vi "Initialize.vi"(8 "error in (no error)":errorcluster, 11 "Socket in":refnum<class "Socket.lvclass">) -> (0 "error out":errorcluster, 3 "Socket out":refnum<class "Socket.lvclass">)   [LabVIEW 2018, in "Socket.lvclass"]
uses:
  Socket.lvclass
  Socket.lvclass/Socket.ctl
  State Machine/State Machine.lvclass
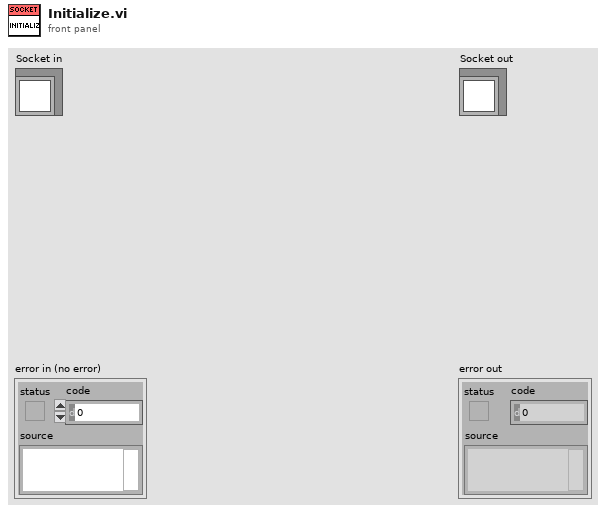
[diagram p1: front panel]
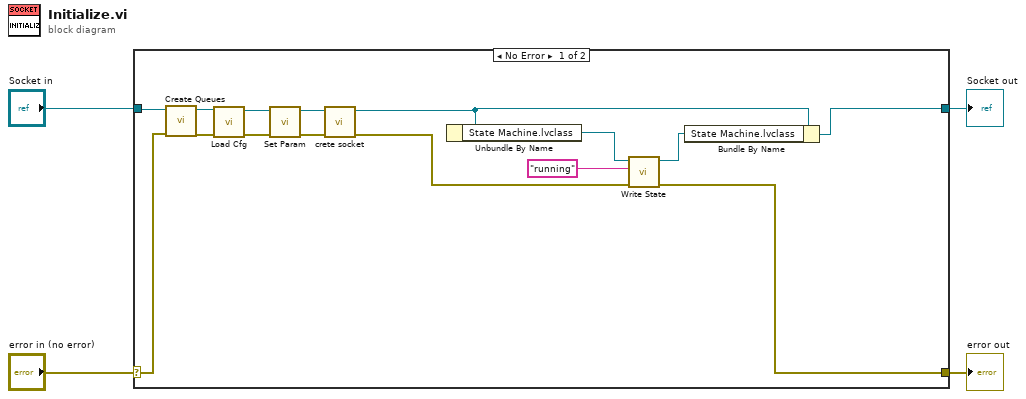
[diagram p0: block diagram]
diagram:
  n1 = case shown="No Error" "error in (no error)" {
    selector: "error in (no error)" -> [w6 w21]
    tunnel: [w9 w21] -> w3
    tunnel: [w19 w20] -> w1
    tunnel: "Socket in" -> [w5 w20]
    frame No Error {
      n2 = call-dynamic "Create Queues.vi"("error in (no error)"=w6, "Socket in"=w5) -> ("error out"=w7:errorcluster, "Socket out"=w8:refnum<class "Socket.lvclass">)  [unwired: 8 in]
      n3 = call-dynamic "Load Cfg.vi"("error in (no error)"=w7, "Socket in"=w8) -> ("error out"=w12:errorcluster, "Socket out"=w15:refnum<class "Socket.lvclass">)  [unwired: 8 in]
      n4 = call-dynamic "Set Param.vi"("error in (no error)"=w12, "Socket in"=w15) -> ("error out"=w11:errorcluster, "Socket out"=w14:refnum<class "Socket.lvclass">)  [unwired: 8 in]
      n5 = call "crete socket.vi"("error in (no error)"=w11, "Socket in"=w14) -> ("error out"=w10:errorcluster, "Socket out"=w13:refnum<class "Socket.lvclass">)  [unwired: 8 in]
      n6 = Unbundle By Name(w13) -> ("State Machine.lvclass"=w17:refnum<class "State Machine.lvclass">)
      n7 = call-dynamic "Write State.vi"("error in (no error)"=w10, "State"="running", "State Machine in"=w17) -> ("error out"=w9:errorcluster, "State Machine out"=w16:refnum<class "State Machine.lvclass">)  [unwired: 7 in]
      n8 = Bundle By Name(cluster=w13, "State Machine.lvclass"=w16) -> (w19:refnum<class "Socket.lvclass">)
    }
    frame Error {
    }
  }
  "error out" <- w3
  "Socket out" <- w1
